vi "Configure Sweep Range.vi"(8 "error in (no error)":errorcluster, 9 "Sweep Range Type (0: Best)":i32(ring) items=["Best", "Fixed"], 10 "Channel (1: Channel 1)":i32(ring)=1 items=["Channel 1"=1, "Channel 2"=2], 11 "VISA resource name":refnum<visa-resource-name>) -> (0 "error out":errorcluster, 3 "VISA resource name out":refnum<visa-resource-name>)   [LabVIEW 2012, in "Keysight B2980 Series.lvlib"]
doc: "Configures the output ranging mode of the sweep output for the specified channel.\n\n<b>Note(s):</b>\nThis VI is only applicable for model B2985A and B2987A."
uses:
  Keysight B2980 Series.lvlib
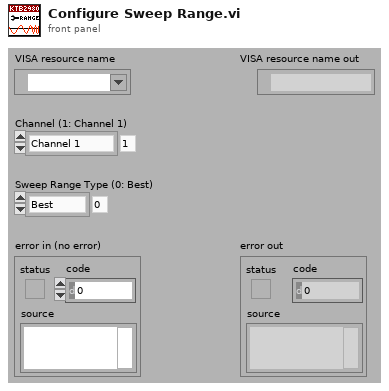
[diagram p1: front panel]
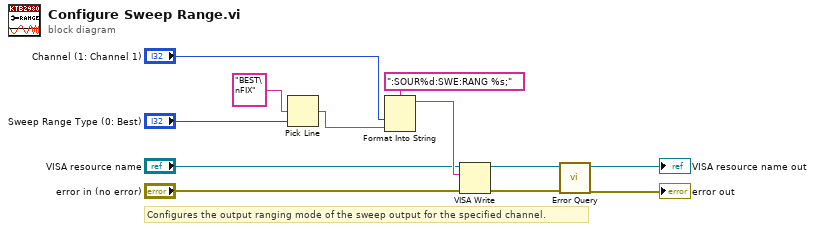
[diagram p0: block diagram]
diagram:
  # "Configures the output ranging mode of the sweep output for the specified channel."
  n1 = Pick Line(multi-line string="BEST\nFIX", line index="Sweep Range Type (0: Best)") -> (output string=w8:string)  [unwired: 1 out]
  n2 = Format Into String(format string=":SOUR%d:SWE:RANG %s;", "Channel (1: Channel 1)", w8) -> (resulting string=w7:string)  [unwired: 2 in, 1 out]
  n3 = VISA Write(VISA resource name="VISA resource name", write buffer=w7, error in (no error)="error in (no error)") -> (VISA resource name out=w4:refnum<visa-resource-name>, error out=w3:errorcluster)  [unwired: 1 out]
  n4 = call "Error Query.vi"("error in (no error)"=w3, "VISA resource name"=w4) -> ("error out"=→"error out":errorcluster, "VISA resource name out"=→"VISA resource name out":refnum<visa-resource-name>)  [unwired: 8 out]
